vi "Find Multiple Enemies.vi"(10 "View":i32[](array[numeric]), 11 "Team Index":i32) -> (2 "Direction":T1[](array[typedef]), 3 "Found Enemy?":bool, 4 "How Many Enemies":i32, 5 "Enemy":i32[](array[numeric]))   [LabVIEW 2020, in "Common.lvlib"]
doc: "Reports whether an enemy is in the vicinity and some information about that enemy."
uses:
  Common.lvlib
  Type Defs/Direction Enum.ctl
  Type Defs/SB Type Defs.lvlib
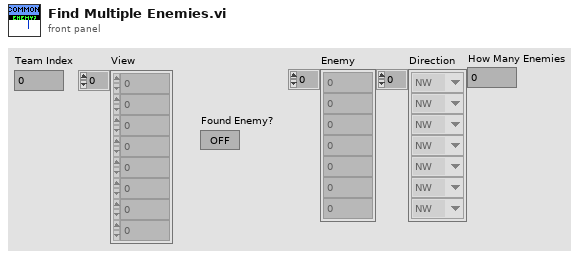
[diagram p1: front panel]
types:
  T1 = typedef "SB Type Defs.lvlib/Direction Enum.ctl" = enum16{"NW", "N", "NE", "E", "SE", "S", "SW", "W"}
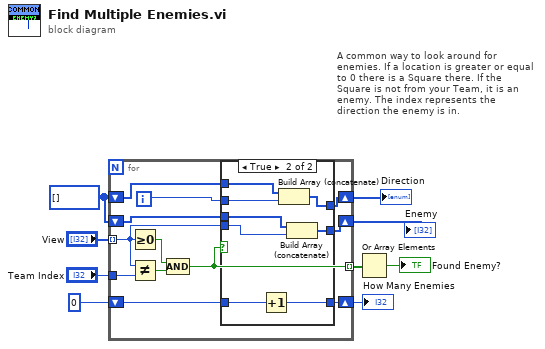
[diagram p0: block diagram]
diagram:
  w4 = i32[] []
  # "A common way to look around for enemies. If a location is greater or equal to 0 there is a Square there. If the Square is not from your Team, it is an enemy. The index represents the direction the enemy is in."
  n1 = for {
    tunnel: "View" -> [w14] mode=indexing
    tunnel: "Team Index" -> [w20]
    tunnel: [w18] -> w6 mode=indexing
    shift-right: [w16] -> w5
    shift-left: w4 -> [w15]
    shift-right: [w13] -> w7
    shift-left: w4 -> [w12]
    shift-right: [w11] -> w1
    shift-left: 0 ("Team Index") -> [w10]
    i -> [w17]
    n2 = Greater Or Equal To 0?(x=w14) -> (x >= 0?=w21:bool)
    n3 = Not Equal?(x=w14, y=w20) -> (x != y?=w19:bool)
    n4 = Compound Arithmetic op=AND(w21, w19) -> (w18:bool)
    n5 = case shown="True" w18 {
      tunnel: w17 -> [_ w32]
      tunnel: [w24 w31] -> w16
      tunnel: w15 -> [w24 w30]
      tunnel: w14 -> [_ w29]
      tunnel: [w23 w28] -> w13
      tunnel: w12 -> [w23 w27]
      tunnel: [w22 w25] -> w11
      tunnel: w10 -> [w22 w26]
      frame False {
      }
      frame True {
        n6 = Increment(x=w26) -> (x+1=w25:i32)
        n7 = Build Array (concatenate)(w30, w32) -> (w31:i32[])
        n8 = Build Array (concatenate)(w27, w29) -> (w28:i32[])
      }
    }
  }
  "Direction" <- w5
  "Enemy" <- w7
  "How Many Enemies" <- w1
  n9 = Or Array Elements(Boolean array=w6) -> (logical OR=→"Found Enemy?":bool)
